vi "Tell Child Init.vi"(7 "Actor in":refnum<class "Actor.lvclass">, 9 "Alias":string, 10 "Msg Attributes":T1) -> (0 "Error out":errorcluster, 1 "Told":bool, 5 "Actor out":refnum<class "Actor.lvclass">)   [LabVIEW 2020, in "jettl.lvlib"]
uses:
  jettl.lvlib
  Actor/Actor.lvclass
  Msg Output/Msg Output.lvclass
  Msg Input/Msg Input.lvclass
  Msg/Msg.lvclass
  Relation.ctl
  Transport/Transport.lvclass
  Msgs.ctl
  Unified Layer.ctl
  Actor Attributes.ctl
  Teller.ctl
  Msg Attributes.ctl
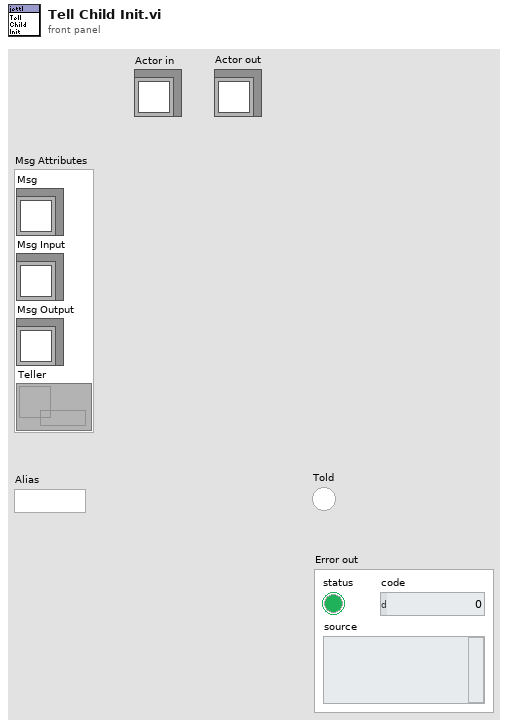
[diagram p1: front panel]
types:
  T1 = typedef "jettl.lvlib/Msg Attributes.ctl" = cluster{"Msg":refnum<class "Msg.lvclass">, "Msg Input":refnum<class "Msg Input.lvclass">, "Msg Output":refnum<class "Msg Output.lvclass">, "Teller":refnum<data-value>}
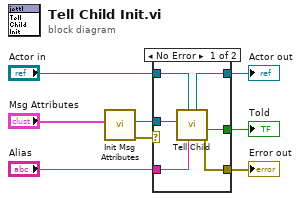
[diagram p0: block diagram]
diagram:
  n1 = call "Init Msg Attributes.vi"("Msg Attributes"="Msg Attributes") -> ("Error out"=w1:errorcluster, "Msg Attributes"=w2:refnum<data-value>)  [unwired: 9 in]
  n2 = case shown="No Error" w1 {
    selector: w1 -> [_ w15]
    tunnel: "Actor in" -> [w14 w16]
    tunnel: [w13 w16] -> w7
    tunnel: [w12 w15] -> w6
    tunnel: "Alias" -> [w11 _]
    tunnel: [w10 _] -> w4
    tunnel: w2 -> [w9 _]
    frame No Error {
      n3 = call "Tell Child.vi"("Alias"=w11, "Actor in"=w14, "Msg Attributes"=w9) -> ("Error out"=w12:errorcluster, "Told"=w10:bool, "Actor out"=w13:refnum<class "Actor.lvclass">)  [unwired: 6 in]
    }
    frame Error {
    }
  }
  "Error out" <- w6
  "Actor out" <- w7
  "Told" <- w4
